vi "WriteSamples.vi"(8 "error in (no error)":errorcluster, 10 "clSampleDataArray":T1, 11 "PmuAnalysis in":refnum<class "PmuAnalysis.lvclass">) -> (0 "error out":errorcluster, 3 "PmuAnalysis out":refnum<class "PmuAnalysis.lvclass">)   [LabVIEW 2014, in "AnalysisPlugins.lvlib" / "PmuAnalysis.lvclass"]
uses:
  PmuAnalysis.lvclass
  AnalysisPluginBaseClass/Typedefs/SampleDataInput.ctl
  AnalysisPluginBaseClass/AnalysisPluginsBase.lvclass/AnalysisPluginsBase.ctl
  AnalysisPluginBaseClass/Accessors/Read SampleDataQueName.vi
  AnalysisPluginBaseClass/AnalysisPluginsBase.lvclass
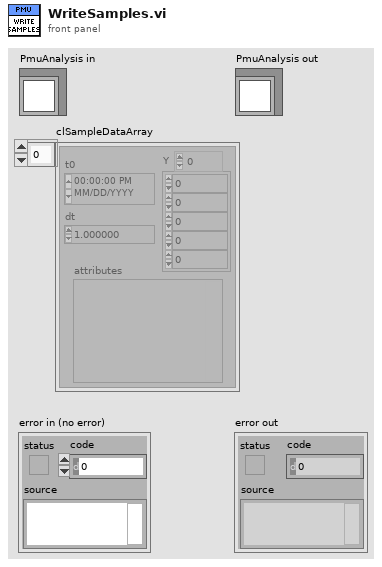
[diagram p1: front panel]
types:
  T1 = typedef "AnalysisPlugins.lvlib/AnalysisPluginsBase.lvclass/SampleDataInput.ctl" = waveform(dbl)[]
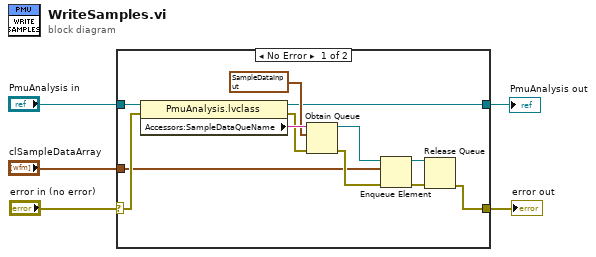
[diagram p0: block diagram]
diagram:
  n1 = case shown="No Error" "error in (no error)" {
    selector: "error in (no error)" -> [w16 w19]
    tunnel: [w6 w19] -> w4
    tunnel: [w7 w18] -> w2
    tunnel: "PmuAnalysis in" -> [w17 w18]
    tunnel: "clSampleDataArray" -> [w8 _]
    frame No Error {
      n2 = property class="PmuAnalysis.lvclass"(reference=w17, error in=w16) -> (reference out=w7:refnum<class "PmuAnalysis.lvclass">, error out=w10:errorcluster, "Accessors:SampleDataQueName"=w11:string)
      n3 = Obtain Queue(name (unnamed)=w11, element data type=T1 [{"t0"=timestamp(0 s since 1904-01-01), "dt"=1.0, "Y"=[]}] ("clSampleDataArray"), error in (no error)=w10) -> (queue out=w12:refnum<queue>, error out=w13:errorcluster)  [unwired: 2 in, 1 out]
      n4 = Enqueue Element(queue=w12, element=w8, error in (no error)=w13) -> (queue out=w15:refnum<queue>, error out=w14:errorcluster)  [unwired: 1 in, 1 out]
      n5 = Release Queue(queue=w15, error in (no error)=w14) -> (error out=w6:errorcluster)  [unwired: 1 in, 2 out]
    }
    frame Error {
    }
  }
  "error out" <- w4
  "PmuAnalysis out" <- w2
